vi "Initialise.vi"(8 "error in (no error)":errorcluster, 10 "Message in":refnum<class "InitialiseMessage.lvclass">, 11 "Chat in":refnum<class "Chat.lvclass">) -> (0 "error out":errorcluster, 3 "Chat out":refnum<class "Chat.lvclass">)   [LabVIEW 2012, in "Chat.lvclass"]
doc: "This method is called when an initialise message is received. It mainly initialises the RabbitMQ connectivity. \n\nOverride this method when your component needs special initialisation (e.g. of software or hardware resources). In that case, don't forget to call the parent for proper implementation. If your component owns subcomponents, they count as resources, so you have to initialise them by calling their own initialise functions"
uses:
  Chat.lvclass
  <vilib>/Distrio/Murmex/InitialiseMessage/InitialiseMessage.lvclass
  <vilib>/Distrio/Murmex/Murmex/Murmex.lvclass
  <vilib>/Distrio/Murmex/InspectMessage/InspectMessage.lvclass
  <vilib>/Distrio/Murmex/Murmex/command_enum.ctl
  <vilib>/Distrio/Murmex/Message/Set triggered-by.vi
panel:
  # "This method is called when the INTIALISE\ntrigger is sent. \n\nOverride this method when your component needs to\nrespond to this trigger. \n\nCall parent for proper implementation"
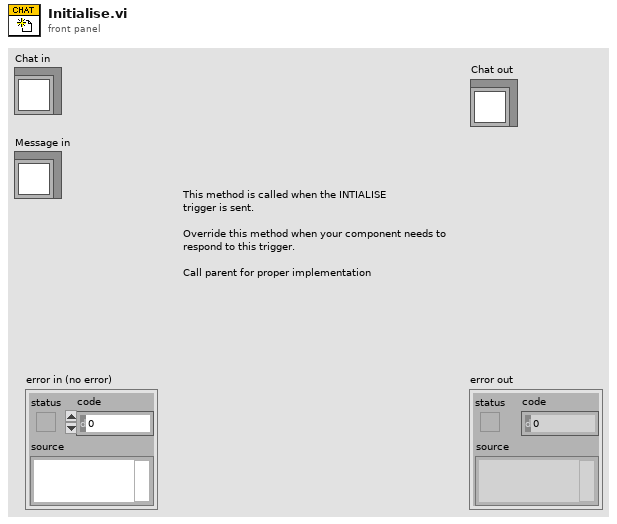
[diagram p1: front panel]
types:
  T1 = typedef "Murmex.lvlib/Murmex.lvclass/command_enum.ctl" = enum16{"null", "initialise", "reset", "terminate", "acknowledge", "update", "inspect", "inform", "proceed", "start", "stop", "fetch", "configure", "generic"}
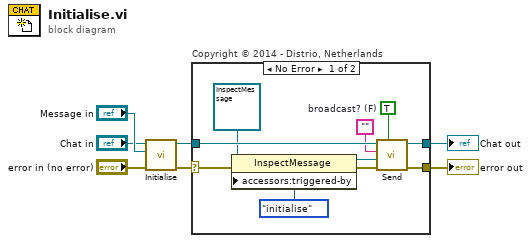
[diagram p0: block diagram]
diagram:
  n1 = call-parent "Initialise.vi"("error in (no error)"="error in (no error)", "Message in"="Message in", "Murmex in"="Chat in") -> ("error out"=w1:errorcluster, "Murmex out"=w3:refnum<class "Chat.lvclass">)  [unwired: 7 in]
  n2 = case "Copyright © 2014 - Distrio, Netherlands" shown="No Error" w1 {
    selector: w1 -> [w10 w19]
    tunnel: [w17 w19] -> w4
    tunnel: w3 -> [w16 w18]
    tunnel: [w15 w18] -> w2
    frame No Error {
      w14 = TRUE  # broadcast? (F)
      n3 = property class="InspectMessage"(reference=refnum<class "InspectMessage.lvclass"> refnum ("Distrio Murmex 1.5:InspectMessage"), error in=w10, "accessors:triggered-by"=command_enum."initialise" ("triggered-by")) -> (reference out=w11:refnum<class "InspectMessage.lvclass">, error out=w9:errorcluster)
      n4 = call <vilib>:"Send.vi"("broadcast? (F)"=w14, "error in (no error)"=w9, "Message"=w11, "recipient"="", "Murmex in"=w16) -> ("error out"=w17:errorcluster, "Murmex out"=w15:refnum<class "Chat.lvclass">)  [unwired: 5 in]
    }
    frame Error {
    }
  }
  "error out" <- w4
  "Chat out" <- w2
